vi "Auto Move Straight.vi"(6 "Target Angle":dbl, 7 "Target Distance":dbl=15.0 format="%#_13g", 8 "Error In":errorcluster, 11 "Refnum's In":T1) -> (0 "Error Out":errorcluster, 3 "Refnum's Out":T1)   [LabVIEW 2016]
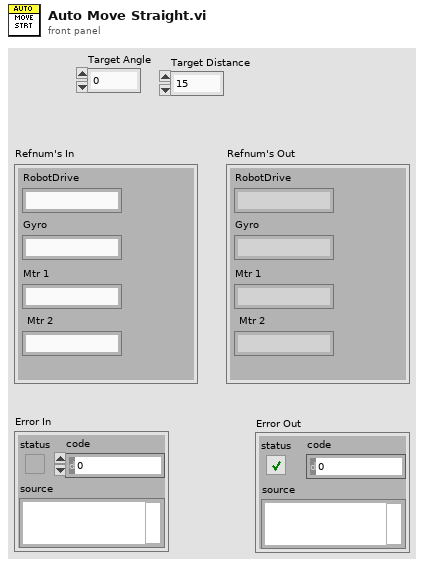
[diagram p1: front panel]
types:
  T1 = cluster{"RobotDrive":string, "Gyro":string, "Mtr 1":string, "Mtr 2":string}
  T2 = typedef "WPI_MotorControlDeviceRef.ctl" = cluster{"DeviceStatus":errorcluster, "Type":T3, "PWM":cluster{"PWM Channel":T4, "DeadBand":T5}, "CAN":cluster{"Device Number":u8, "SetOutput VI Ref":variant, "GetOutput VI Ref":variant, "Enable VI Ref":variant, "Disable VI Ref":variant, "Data":variant}, "Invert":bool}
  T3 = typedef "WPI_MotorControlType.ctl" = enum16{"PWM", "CAN"}
  T4 = typedef "FPGA_DIOPWMChannel.ctl" = enum8{"PWM 0", "PWM 1", "PWM 2", "PWM 3", "PWM 4", "PWM 5", "PWM 6", "PWM 7", "PWM 8", "PWM 9", "PWM MXP 0", "PWM MXP 1", "PWM MXP 2", "PWM MXP 3", "PWM MXP 4", "PWM MXP 5", "PWM MXP 6", "PWM MXP 7", "PWM MXP 8", "PWM MXP 9", "Invalid"}
  T5 = typedef "WPI_PWMDeadband.ctl" = cluster{"Name":string, "maxPositivePwm":i32, "minPositivePwm":i32, "centerPwm":i32, "maxNegativePwm":i32, "minNegativePwm":i32, "angularRange":u16}
  T6 = typedef "WPI_GyroDevRef.ctl" = cluster{"DevStatus":errorcluster, "Analog Channel":T7, "Offset":dbl, "Gain (VoltsPerDegree/Second)":dbl, "Gyro Type":enum16{"Analog", "XRS450"}, "Handle":i32, "SPI Bus":T8, "Device Found":bool, "Sample Rate":dbl, "Calibrate On Open":bool}
  T7 = typedef "FPGA_AIChannel.ctl" = enum8{"AI 0", "AI 1", "AI 2", "AI 3", "AI MXP 0", "AI MXP 1", "AI MXP 2", "AI MXP 3", "Invalid"}
  T8 = typedef "spi_bus.ctl" = enum16{"SPI On-Board, CS0", "SPI On-Board, CS1", "SPI On-Board, CS2", "SPI On-Board, CS3", "SPI MXP", "Invalid"}
  T9 = typedef "WPI_CANTalonSRX_GlobalStatus.ctl" = cluster{"Applied Throttle":dbl, "Module Enabled":bool, "CAN Error":errorcluster, "Closed Loop Error":dbl, "Forward Limit Switch Closed":bool, "Reverse Limit Switch Closed":bool, "Sensor Position":dbl, "Sensor Velocity":dbl, "Current":dbl, "Sticky Fault - Over Temp":bool, "Sticky Fault - Under Voltage":bool, "Sticky Fault - Forward Limit":bool, "Sticky Fault - Reverse Limit":bool, "Sticky Fault - Forward Soft Limit":bool, "Sticky Fault - Reverse Soft Limit":bool, "Brake is Enabled":bool, "Encoder Position":dbl, "Encoder Velocity":dbl, "Encoder Index Count":dbl, "Encoder A Pin State":bool, "Encoder B Pin State":bool, "Encoder Index Pin State":bool, "Analog In":dbl, "Analog In Velocity":dbl, "Temperature (C)":dbl, "Battery Voltage":dbl, "Control 5 Is Supported":bool, "Current Profile Slot Select":dbl, "Pos Div 8":bool, "Vel Div 4":bool, "Pulse Width Position":i32, "Pulse Width Velocity":i32, "Pulse Width Rise To Rise (us)":i32, "Pulse Width Rise To Fall (us)":i32, "Mot Prof Active Is Under Run":bool, "Mot Prof Active Has Under Run":bool, "Mot Prof Active Is Last":bool, "Mot Prof Active Velocity Only":bool, "Mot Prof Active Is Valid":bool, "Mot Prof Buffer Is Full":bool, "Mot Prof Active Profile Slot Select":i32, "Mot Prof NextID":i32, "Mot Prof Count":i32, "Mot Prof Active Velocity":dbl, "Mot Prof Active Position":dbl, "Mot Prof Output Enable":i32}
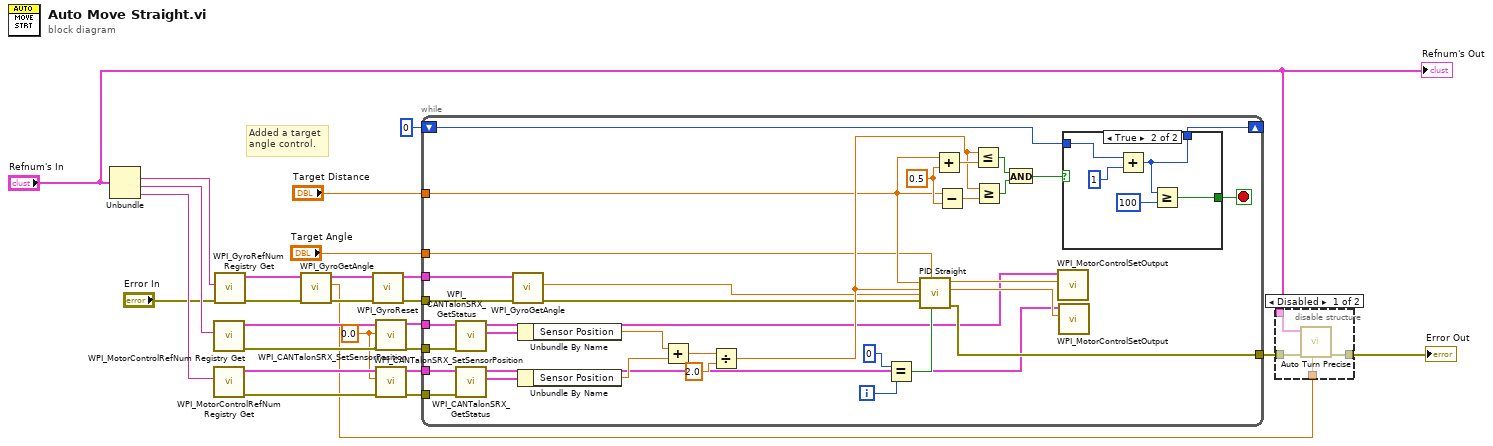
[diagram p0: block diagram]
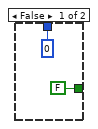
[diagram p3: hidden frame]
diagram:
  w16 = 0.0 ("New Sensor Position")
  # "Added a target\nangle control."
  n1 = Unbundle("Refnum's In") -> ("Gyro"=w12:string, "Mtr 1"=w11:string, "Mtr 2"=w10:string)  [unwired: 1 out]
  n2 = call <vilib>:"WPI_MotorControlRefNum Registry Get.vi"("refnum name"=w11) -> ("error out"=w19:errorcluster, "MotorControlDevRef"=w20:T2)  [unwired: 9 in]
  n3 = call <vilib>:"WPI_MotorControlRefNum Registry Get.vi"("refnum name"=w10) -> ("error out"=w22:errorcluster, "MotorControlDevRef"=w21:T2)  [unwired: 9 in]
  n4 = call <vilib>:"WPI_GyroRefNum Registry Get.vi"("error in (no error)"="Error In", "refnum name"=w12) -> ("error out"=w3:errorcluster, "GyroDevRef"=w4:T6)  [unwired: 8 in]
  n5 = call <vilib>:"WPI_GyroGetAngle.vi"("error in"=w3, "GyroDevRef"=w4) -> ("error out"=w25:errorcluster, "Angle"=w5:dbl, "GyroDevRef"=w26:T6)  [unwired: 5 in, 2 out]
  n6 = call <vilib>:"WPI_GyroReset.vi"("error in"=w25, "GyroDevRef"=w26) -> ("error out"=w24:errorcluster, "GyroDevRef"=w23:T6)  [unwired: 8 in]
  n7 = call <vilib>:"WPI_CANTalonSRX_SetSensorPosition.vi"("error in (no error)"=w19, "New Sensor Position"=w16, "CAN Talon SRX Ref"=w20) -> ("error out"=w15:errorcluster, "CAN Talon SRX Ref"=w14:T2)  [unwired: 7 in]
  n8 = call <vilib>:"WPI_CANTalonSRX_SetSensorPosition.vi"("error in (no error)"=w22, "New Sensor Position"=w16, "CAN Talon SRX Ref"=w21) -> ("error out"=w17:errorcluster, "CAN Talon SRX Ref"=w18:T2)  [unwired: 7 in]
  n9 = while {
    tunnel: w23 -> [w54]
    tunnel: w24 -> [w53]
    tunnel: w14 -> [w52]
    tunnel: w15 -> [w51]
    tunnel: w18 -> [w50]
    tunnel: w17 -> [w49]
    shift-right: [w41] -> _
    shift-left: 0 -> [w40]
    tunnel: "Target Distance" -> [w28]
    tunnel: [w36] -> w9
    tunnel: "Target Angle" -> [w27]
    i -> [w60]
    stop <- w35 stop-if-true
    w48 = 0.5 ("y")
    n10 = call <vilib>:"WPI_CANTalonSRX_GetStatus.vi"("error in (no error)"=w51, "CAN Talon SRX Ref"=w52) -> ("Talon SRX Status"=w55:T9, "CAN Talon SRX Ref"=w29:T2)  [unwired: 7 in, 1 out]
    n11 = call <vilib>:"WPI_CANTalonSRX_GetStatus.vi"("error in (no error)"=w49, "CAN Talon SRX Ref"=w50) -> ("Talon SRX Status"=w56:T9, "CAN Talon SRX Ref"=w30:T2)  [unwired: 7 in, 1 out]
    n12 = call <vilib>:"WPI_GyroGetAngle.vi"("error in"=w53, "GyroDevRef"=w54) -> ("error out"=w37:errorcluster, "Angle"=w39:dbl)  [unwired: 5 in, 3 out]
    n13 = Unbundle By Name(w55) -> ("Sensor Position"=w34:dbl)
    n14 = Unbundle By Name(w56) -> ("Sensor Position"=w33:dbl)
    n15 = Add(x=w34, y=w33) -> (x+y=w57:dbl)
    n16 = Divide(x=w57, y=2.0) -> (x/y=w46:dbl)
    n17 = Equal?(x=0, y=w60) -> (x = y?=w38:bool)
    n18 = call "PID Straight.vi"("Reinitialize"=w38, "Target Angle"=w27, "Error In"=w37, "Gyro Angle"=w39, "Current Distance"=w46, "Target Distance"=w28) -> ("Error Out"=w36:errorcluster, "Right Power"=w31:dbl, "Left Power"=w32:dbl)  [unwired: 3 in]
    n19 = Add(x=w28, y=w48) -> (x+y=w47:dbl)
    n20 = Subtract(x=w28, y=w48) -> (x-y=w45:dbl)
    n21 = Less Or Equal?(x=w46, y=w47) -> (x <= y?=w44:bool)
    n22 = Greater Or Equal?(x=w46, y=w45) -> (x >= y?=w43:bool)
    n23 = And(x=w44, y=w43) -> (x .and. y?=w42:bool)
    n24 = call <vilib>:"WPI_MotorControlSetOutput.vi"("Output"=w32, "MotorControlDevRef"=w29) -> ()  [unwired: 7 in, 3 out]
    n25 = call <vilib>:"WPI_MotorControlSetOutput.vi"("Output"=w31, "MotorControlDevRef"=w30) -> ()  [unwired: 7 in, 3 out]
    n26 = case shown="True" w42 {
      tunnel: w40 -> [_ w66]
      tunnel: [0 w65] -> w41
      tunnel: [FALSE w63] -> w35
      frame False {
      }
      frame True {
        n27 = Add(x=w66, y=1) -> (x+y=w65:i32)
        n28 = Greater Or Equal?(x=w65, y=100) -> (x >= y?=w63:bool)
      }
    }
  }
  n29 = disable-structure shown="Disabled" {
    disable-tunnel: w9 -> [w71 _]
    disable-tunnel: [w70 _] -> w7
    disable-tunnel: "Refnum's In" -> [w69 _]
    disable-tunnel: w5 -> [w68 _]
    frame Disabled {
      n30 = call "Auto Turn Precise.vi"("Target Distance"=w68, "Error In"=w71, "Refnum's In"=w69) -> ("Error Out"=w70:errorcluster)  [unwired: 7 in, 1 out]
    }
    frame Enabled {
    }
  }
  "Error Out" <- w7
  "Refnum's Out" <- "Refnum's In"
